vi "DSF.Engine.Memory.BufferPool.Obtain Buffer.vi"(8 "error in (no error)":errorcluster, 9 "timeout ms (0)":i32 format="%d ms", 11 "BufferPool in":refnum<class "DSF.Engine.Memory.BufferPool.lvclass">) -> (0 "error out":errorcluster, 1 "timed out?":bool, 2 "Buffer":refnum<class "DSF.Engine.Memory.Buffer.lvclass">, 3 "BufferPool out":refnum<class "DSF.Engine.Memory.BufferPool.lvclass">)   [LabVIEW 2016, in "DSF.Engine.lvlib" / "DSF.Engine.Memory.BufferPool.lvclass"]
uses:
  BufferPool/DSF.Engine.Memory.BufferPool.lvclass
  Buffer/DSF.Engine.Memory.Buffer.lvclass
  BufferPool/DSF.Engine.Memory.BufferPool.lvclass/DSF.Engine.Memory.BufferPool.ctl
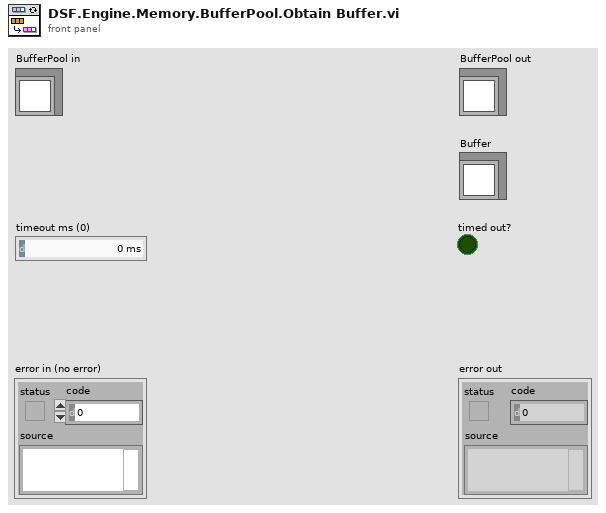
[diagram p1: front panel]
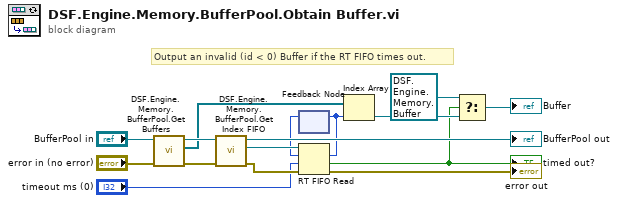
[diagram p0: block diagram]
diagram:
  # "Output an invalid (id < 0) Buffer if the RT FIFO times out."
  n1 = call "DSF.Engine.Memory.BufferPool.Get Buffers.vi"("error in (no error)"="error in (no error)", "BufferPool in"="BufferPool in") -> ("error out"=w10:errorcluster, "Buffers"=w9:refnum<class "DSF.Engine.Memory.Buffer.lvclass">[], "BufferPool out"=w11:refnum<class "DSF.Engine.Memory.BufferPool.lvclass">)  [unwired: 7 in]
  n2 = call "DSF.Engine.Memory.BufferPool.Get Index FIFO.vi"("error in (no error)"=w10, "BufferPool in"=w11) -> ("error out"=w15:errorcluster, "Index FIFO"=w16:refnum<k33>, "BufferPool out"=→"BufferPool out":refnum<class "DSF.Engine.Memory.BufferPool.lvclass">)  [unwired: 7 in]
  n3 = feedback #1() -> (w2:i32)  [unwired: 1 in]
  n4 = RT FIFO Read(0:w16, 1:w2, 2:"timeout ms (0)", 3:w15) -> (9:w1:i32, 10:w3:bool, 11:→"error out":errorcluster)  [unwired: 2 out]
  "timed out?" <- w3
  n5 = feedback-in #1(w1) -> ()
  n6 = Index Array(array=w9, index=w1) -> (element=w6:refnum<class "DSF.Engine.Memory.Buffer.lvclass">)
  n7 = Select(t=refnum<class "DSF.Engine.Memory.Buffer.lvclass"> refnum, s=w3, f=w6) -> (s? t:f=→"Buffer":refnum<class "DSF.Engine.Memory.Buffer.lvclass">)
